vi "Send Current.vi"(8 "error in (no error)":errorcluster, 10 "Current (4 mA)":dbl=4.0, 11 "VISA resource name":refnum<visa-resource-name>) -> (0 "error out":errorcluster, 3 "VISA resource name out":refnum<visa-resource-name>)   [LabVIEW 2023, in "Fluke Molbox 1 Plus.lvlib"]
doc: "Send a current to the MFC if in current mode. The optional MFC interface can set a current for an MFC. the molbox1+ must be in current mode before this can be done. The data is always in \"mA\". This command does not change the regulation mode target for the MFC."
uses:
  Fluke Molbox 1 Plus.lvlib
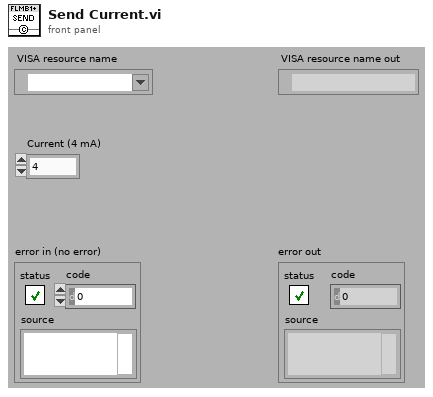
[diagram p1: front panel]
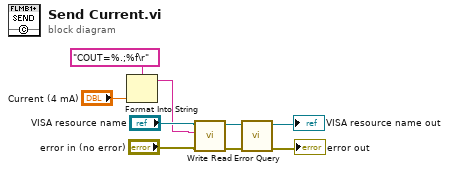
[diagram p0: block diagram]
diagram:
  n1 = Format Into String(format string="COUT=%.;%f\r", "Current (4 mA)") -> (resulting string=w5:string)  [unwired: 2 in, 1 out]
  n2 = call "Write Read.vi"("error in (no error)"="error in (no error)", "Write String"=w5, "VISA resource name"="VISA resource name") -> ("error out"=w3:errorcluster, "VISA resource name out"=w4:refnum<visa-resource-name>)  [unwired: 6 in, 1 out]
  n3 = call "Error Query.vi"("error in (no error)"=w3, "VISA resource name"=w4) -> ("error out"=→"error out":errorcluster, "VISA resource name out"=→"VISA resource name out":refnum<visa-resource-name>)  [unwired: 6 in, 2 out]
